vi "testOnlineMap2.vi"() -> ()   [LabVIEW 2011]
uses:
  <vilib>/vision/NI_Vision_Development_Module.lvlib
panel:
  out "Image 5":T1(plugin-control)
  out "Image 4":T1(plugin-control)
  out "Image 3":T1(plugin-control)
  out "Image 2":T1(plugin-control)
  out "Image":T1(plugin-control)
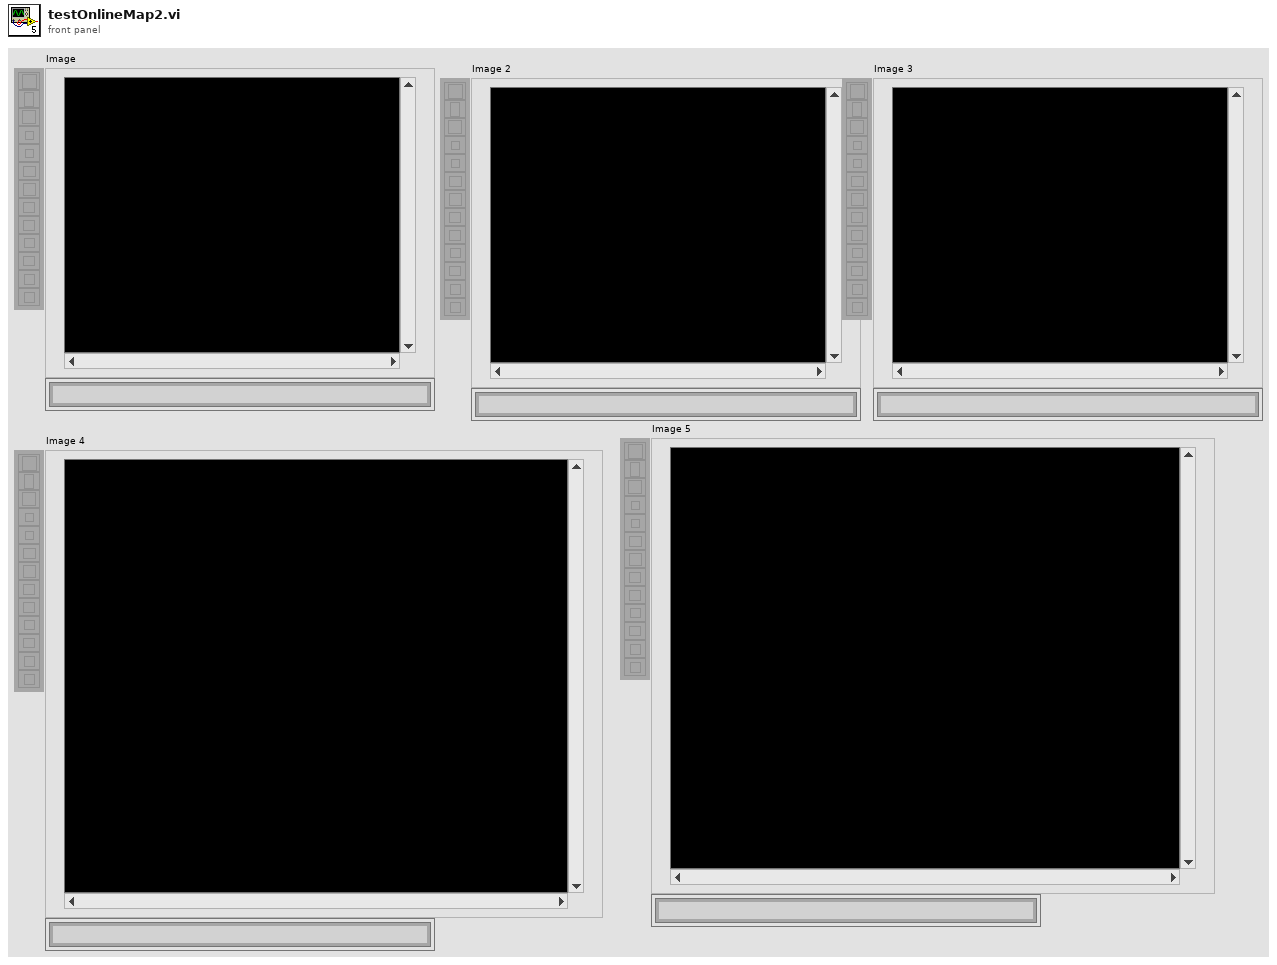
[diagram p1: front panel]
types:
  T1 = typedef "IMAQ Image.ctl" = refnum<image>
  T2 = cluster{"frame_zero_0":i32, "frame_zero_1":i32, "frame_0":i32, "frame_1":i32}
  T3 = typedef "Image Type" = u32
  T4 = cluster{"Mean Value":sgl, "Standard Variation":sgl, "Minimal Value":sgl, "Maximal Value":sgl, "Area (calibrated)":sgl, "Area (pixels)":u32, "%":sgl, "Calibration Valid":bool}
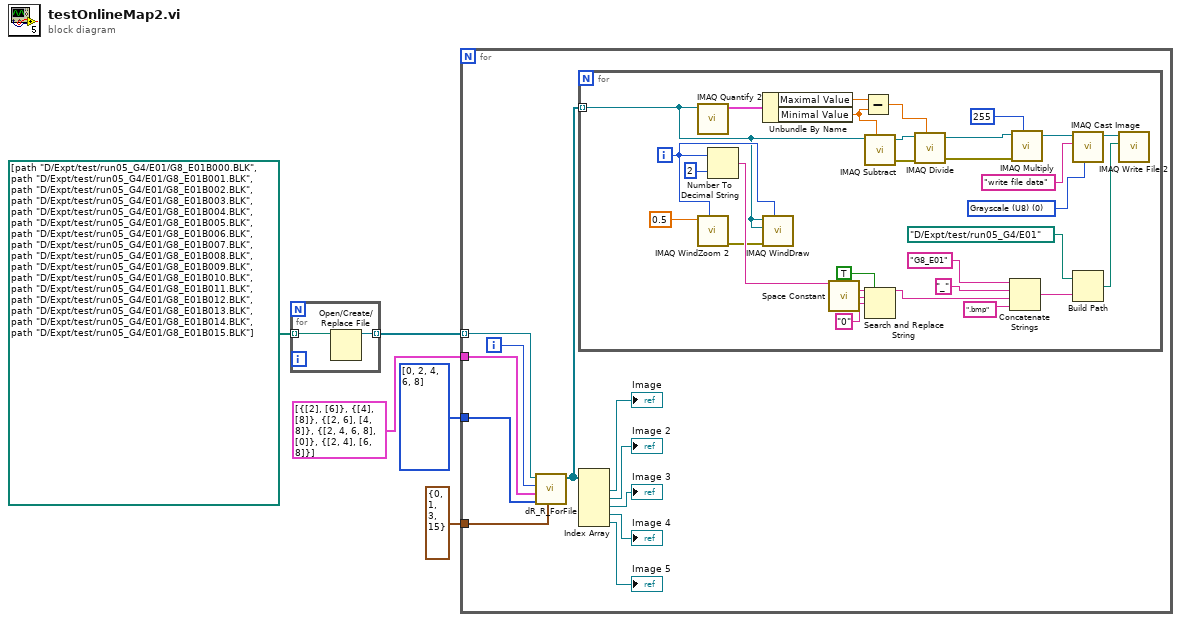
[diagram p0: block diagram]
diagram:
  n1 = for {
    tunnel: path[] [path "D:/Expt/test/run05_G4/E01/G8_E01B000.BLK", path "D:/Expt/test/run05_G4/E01/G8_E01B001.BLK", path "D:/Expt/test/run05_G4/E01/G8_E01B002.BLK", path "D:/Expt/test/run05_G4/E01/G8_E01B003.BLK", path "D:/Expt/test/run05_G4/E01/G8_E01B004.BLK", path "D:/Expt/test/run05_G4/E01/G8_E01B005.BLK", path "D:/Expt/test/run05_G4/E01/G8_E01B006.BLK", path "D:/Expt/test/run05_G4/E01/G8_E01B007.BLK", path "D:/Expt/test/run05_G4/E01/G8_E01B008.BLK", path "D:/Expt/test/run05_G4/E01/G8_E01B009.BLK", path "D:/Expt/test/run05_G4/E01/G8_E01B010.BLK", path "D:/Expt/test/run05_G4/E01/G8_E01B011.BLK", path "D:/Expt/test/run05_G4/E01/G8_E01B012.BLK", path "D:/Expt/test/run05_G4/E01/G8_E01B013.BLK", path "D:/Expt/test/run05_G4/E01/G8_E01B014.BLK", path "D:/Expt/test/run05_G4/E01/G8_E01B015.BLK"] ("数组") -> [w7] mode=indexing
    tunnel: [w6] -> w1 mode=indexing
    n2 = Open/Create/Replace File(file path (use dialog)=w7) -> (refnum out=w6:refnum<file>)  [unwired: 5 in, 2 out]
  }
  n3 = for {
    tunnel: cluster{"数组 1":i32[], "数组 2":i32[]}[] [{"数组 1"=[2], "数组 2"=[6]}, {"数组 1"=[4], "数组 2"=[8]}, {"数组 1"=[2, 6], "数组 2"=[4, 8]}, {"数组 1"=[2, 4, 6, 8], "数组 2"=[0]}, {"数组 1"=[2, 4], "数组 2"=[6, 8]}] ("OnlineMap") -> [w18]
    tunnel: u8[] [0, 2, 4, 6, 8] ("stim ID") -> [w17]
    tunnel: T2 {"frame_zero_0"=0, "frame_zero_1"=1, "frame_0"=3, "frame_1"=15} ("DR/R parameter") -> [w16]
    tunnel: w1 -> [w15] mode=indexing
    i -> [w14]
    n4 = call "dR_R_ForFile.vi"("DR/R parameter"=w16, "stim ID"=w17, "OnlineMap"=w18, "blkIndex"=w14, "BlkFile"=w15) -> ("onLineMapOutput"=w8:T1[])  [unwired: 6 in]
    n5 = for {
      tunnel: w8 -> [w21] mode=indexing
      i -> [w47]
      w35 = T3 0 items=["Grayscale (U8)", "Grayscale (I16)", "Grayscale (SGL)", "Complex (CSG)", "RGB (U32)", "HSL (U32)", "RGB (U64)", "Grayscale (U16)"] ("Image Type")
      n6 = call "IMAQ Quantify 2"("Image"=w21) -> ("Global Report"=w33:T4)  [unwired: 8 in, 2 out]
      n7 = call "IMAQ WindZoom 2"("Window Number (0...15)"=w47, "Zoom Factor"=sgl 0.5) -> ("error out"=w31:errorcluster)  [unwired: 6 in, 3 out]
      n8 = Number To Decimal String(number=w47, width (-)=i16 2 ("宽度(-)")) -> (decimal integer string=w44:string)
      n9 = Unbundle By Name(w33) -> ("Maximal Value"=w32:sgl, "Minimal Value"=w30:sgl)
      n10 = call "IMAQ WindDraw"("Window Number (0...15)"=w47, "error in (no error)"=w31, "Title"=w21, "Image"=w21) -> ()  [unwired: 6 in, 2 out]
      n11 = call <vilib>:"Space Constant.vi"() -> ("String"=w43:string)
      n12 = Subtract(x=w32, y=w30) -> (x-y=w27:sgl)
      n13 = call "IMAQ Subtract"("Image Src A"=w21, "Constant"=w30) -> ("Image Dst Out"=w28:T1, "error out"=w29:errorcluster)  [unwired: 5 in]
      n14 = Search and Replace String(replace all?=TRUE ("替换全部？(F)"), input string=w44, search string=w43, replace string="0" ("替换字符串(\"\")")) -> (result string=w39:string)  [unwired: 4 in, 3 out]
      n15 = call "IMAQ Divide"("Image Src A"=w28, "Constant"=w27, "error in (no error)"=w29) -> ("Image Dst Out"=w25:T1, "error out"=w26:errorcluster)  [unwired: 4 in]
      n16 = Concatenate Strings("G8_E01" ("文件名"), "_" ("字符串"), w39, ".bmp" ("字符串")) -> (w37:string)
      n17 = call "IMAQ Multiply"("Image Src A"=w25, "Constant"=255, "error in (no error)"=w26) -> ("Image Dst Out"=w23:T1)  [unwired: 4 in, 1 out]
      n18 = call "IMAQ Cast Image"("Image Type"=w35, "Image Dst"="write file data" ("替换字符串(\"\")"), "Image Src"=w23) -> ("Image Dst Out"=w34:T1)  [unwired: 7 in, 1 out]
      n19 = Build Path(base path=path "D:/Expt/test/run05_G4/E01" ("Blk目录"), name or relative path=w37) -> (appended path=w36:path)
      n20 = call-poly "IMAQ Write File 2"("File Path"=w36, "Image"=w34) -> ()  [unwired: 8 in, 2 out]
    }
    n21 = Index Array(array=w8) -> (element #1=→"Image":T1, element #2=→"Image 2":T1, element #3=→"Image 3":T1, element #4=→"Image 4":T1, element #5=→"Image 5":T1)  [unwired: 5 in]
  }
